vi "Wiimote unregister for extension events.vi"(8 "error in":errorcluster, 11 "LV WiiMote Interface In":T1) -> (0 "error out":errorcluster, 3 "LV WiiMote Interface out":T1)   [LabVIEW 2012, in "LV Wiimote Interface.lvclass"]
uses:
  LV Wiimote Interface.lvclass
  Controls/LV Wiimote Interface.ctl
  LV Wiimote Interface.lvclass/LV Wiimote Interface.ctl
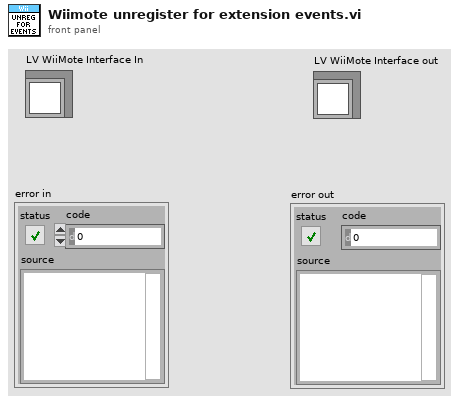
[diagram p1: front panel]
types:
  T1 = typedef "LV Wiimote Interface.ctl" = refnum<class "LV Wiimote Interface.lvclass">
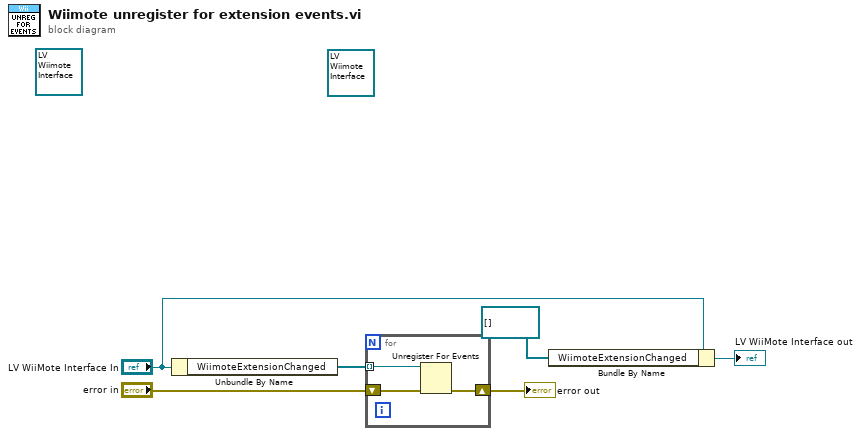
[diagram p0: block diagram]
diagram:
  (unwired) T1 refnum ("LV WiiMote Interface In")
  (unwired) T1 refnum ("LV WiiMote Interface out")
  n1 = Unbundle By Name("LV WiiMote Interface In") -> ("WiimoteExtensionChanged"=w6:refnum<k27>[])
  n2 = for {
    tunnel: w6 -> [w9] mode=indexing
    shift-right: [w7] -> w4
    shift-left: "error in" -> [w8]
    n3 = Unregister For Events(event registration refnum=w9, error in=w8) -> (error out=w7:errorcluster)
  }
  "error out" <- w4
  n4 = Bundle By Name(cluster="LV WiiMote Interface In", "WiimoteExtensionChanged"=refnum<k27>[] []) -> (→"LV WiiMote Interface out":T1)
